vi "Point to Oval.vi"(0 "Image In":T1, 1 "Point":cluster{"X \nX":dbl, "Y":dbl}, 2 "Size":dbl) -> (3 "Image Out":T1(plugin-control))   [LabVIEW 2015]
doc: "This takes only one point and makes it an oval. I just took the \"Points to Oval\" program and removed the array stuff and the loop. It takes only one point."
uses:
  <vilib>/vision/Image Controls.llb/IMAQ Image.ctl
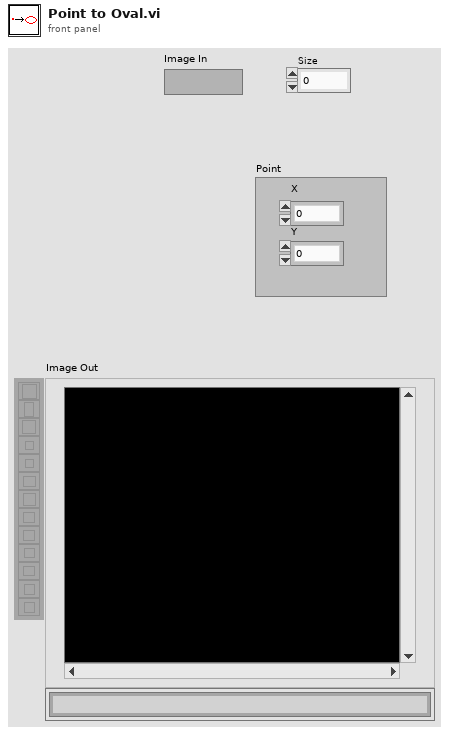
[diagram p1: front panel]
types:
  T1 = typedef "IMAQ Image.ctl" = refnum<image>
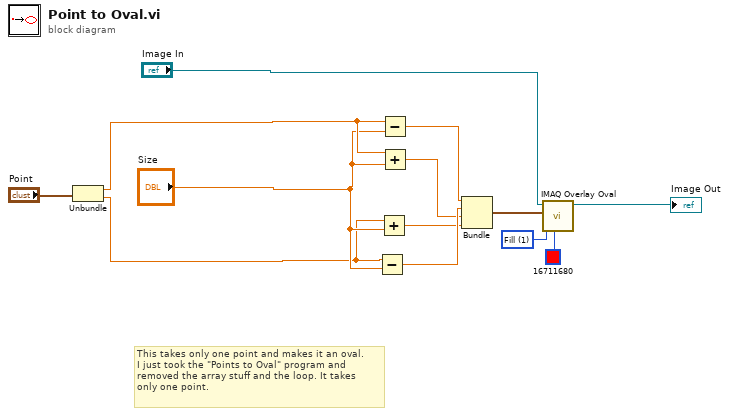
[diagram p0: block diagram]
diagram:
  w5 = u32 1 items=["Frame", "Fill"] ("Drawing Mode (Frame)")
  # "This takes only one point and makes it an oval.\nI just took the \"Points to Oval\" program and \nremoved the array stuff and the loop. It takes\nonly one point."
  n1 = Unbundle("Point") -> ("X \nX"=w4:dbl, "Y"=w1:dbl)
  n2 = Subtract(x=w1, y="Size") -> (x-y=w11:dbl)
  n3 = Add(x=w1, y="Size") -> (x+y=w9:dbl)
  n4 = Subtract(x=w4, y="Size") -> (x-y=w12:dbl)
  n5 = Add(x=w4, y="Size") -> (x+y=w10:dbl)
  n6 = Bundle(w12, w11, w10, w9) -> (w8:cluster{dbl, dbl, dbl, dbl})  [unwired: 1 in]
  n7 = call "IMAQ Overlay Oval"("Color"=u32 16711680, "Drawing Mode (Frame)"=w5, "Bounding Rectangle"=w8, "Image"="Image In") -> ("Image Out"=→"Image Out":T1)  [unwired: 6 in, 1 out]
